vi "Test Compare Equal 1el String Arrays.vi"(8 "error in (no error)":errorcluster, 11 "Comparison Test Double in":refnum<class "Comparison Test Double.lvclass">) -> (0 "error out":errorcluster, 3 "Comparison Test Double out":refnum<class "Comparison Test Double.lvclass">)   [LabVIEW 2020, in "Comparison Test Double.lvclass"]
uses:
  Comparison Test Double.lvclass
  C:/git/astemes-lunit/source/LUnit Test Case.lvclass
  source/LUnit Test Case.lvclass/LUnit Test Case.ctl
  2e376786-aa96-4976-8152-b36927c13d03.vi
  source/Core/LUnit Test Case/Private/Append Pass Result.vi
  source/Core/LUnit Test Case/Private/Append Fail Result.vi
  2e376786-aa96-4976-8152-b36927c13d03.vi/9c5d11cd-9439-4240-a1ee-d9baace9c924.vi
  source/Core/LUnit Test Case/Private/Run In UI.vi
  <vilib>/Utility/error.llb/Clear Errors.vi
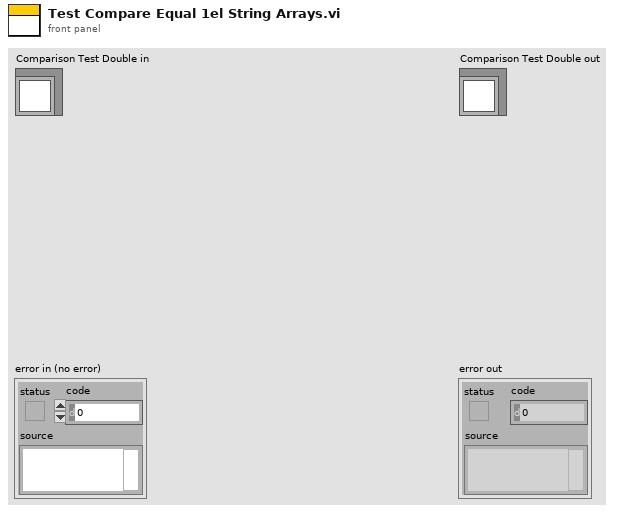
[diagram p1: front panel]
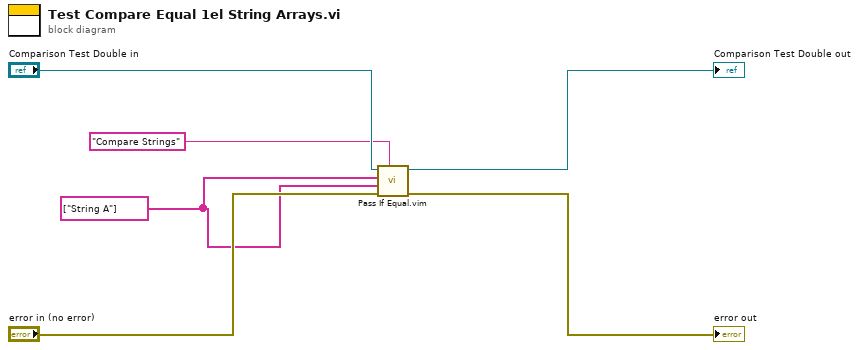
[diagram p0: block diagram]
diagram:
  w1 = string[] ["String A"]
  n1 = call "Pass If Equal.vim"("Description"="Compare Strings", "error in (no error)"="error in (no error)", "Actual"=w1, "Expected"=w1, "LUnit Test Case In"="Comparison Test Double in") -> ("error out"=→"error out":errorcluster, "LUnit Test Case Out"=→"Comparison Test Double out":refnum<class "Comparison Test Double.lvclass">)  [unwired: 5 in]
